vi "Get Color Icon from Caller.vi"() -> (3 "color":T1)   [LabVIEW 2021]
uses:
  <vilib>/picture/picture.llb/imagedata.ctl
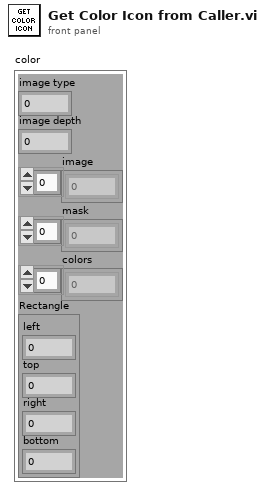
[diagram p1: front panel]
types:
  T1 = typedef "imagedata.ctl" = cluster{"image type":i32, "image depth":i32, "image":u8[], "mask":u8[], "colors":u32[], "Rectangle":cluster{"left":i16, "top":i16, "right":i16, "bottom":i16}}
  T2 = typedef "Who Invoked Icon Editor.ctl" = cluster{"Icon Editor Invoker Type":T3, "App Refnum of Invoker":refnum<vi>, "Qualified Name of Invoker":string, "Path to Invoker":path}
  T3 = typedef "Icon Editor Invoker Type.ctl" = enum32{"Unknown Icon Source", "VI Icon", "Library Icon (any library type)", "Palette icon", "Icon from App Method"}
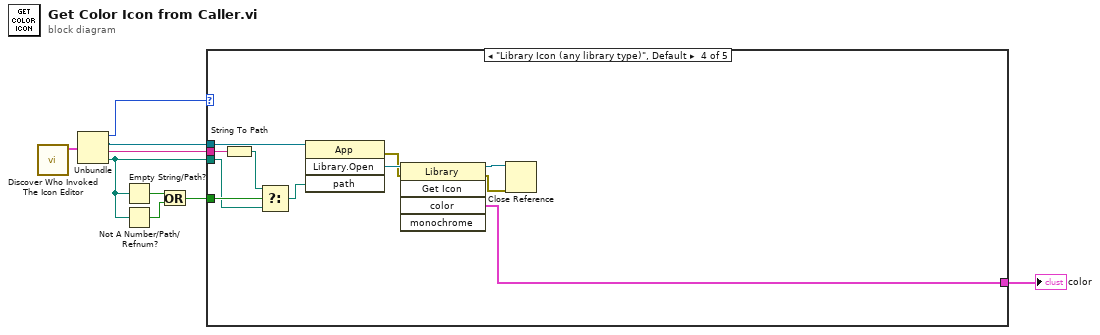
[diagram p0: block diagram]
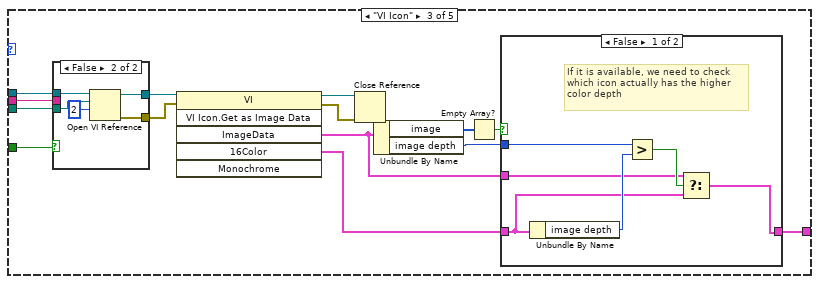
[diagram p4: hidden frame]
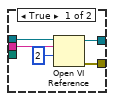
[diagram p6: hidden frame]
diagram:
  n1 = call <resource>:"Discover Who Invoked The Icon Editor.vi"() -> ("Who Invoked The Icon Editor?"=w9:T2)  [unwired: 11 out]
  n2 = Unbundle(w9) -> ("Icon Editor Invoker Type"=w7:T3, "App Refnum of Invoker"=w8:refnum<vi>, "Qualified Name of Invoker"=w3:string, "Path to Invoker"=w2:path)
  n3 = Empty String/Path?(string/path=w2) -> (empty?=w6:bool)
  n4 = Not A Number/Path/Refnum?(number/path/refnum=w2) -> (NaN/Path/Refnum?=w5:bool)
  n5 = Or(x=w6, y=w5) -> (x .or. y?=w4:bool)
  n6 = case shown="\"Library Icon (any library type)\", Default" w7 {
    tunnel: w8 -> [_ _ w21 w49 _]
    tunnel: w3 -> [_ _ w19 w45 _]
    tunnel: w2 -> [_ _ w18 w46 _]
    tunnel: w4 -> [_ _ w20 w47 _]
    tunnel: [_ _ w13 w41 _] -> w1
    frame "Unknown Icon Source" {
    }
    frame "Icon from App Method" {
    }
    frame "VI Icon" {
      n7 = case shown="False" w20 {
        tunnel: [w35 w40] -> w23
        tunnel: [w34 w39] -> w22
        tunnel: w21 -> [w33 w38]
        tunnel: w19 -> [w32 _]
        tunnel: w18 -> [_ w37]
        frame True {
          n8 = Open VI Reference(application reference (local)=w33, vi path=w32, options=2) -> (vi reference=w35:refnum<vi>, error out=w34:errorcluster)  [unwired: 1 in, 2 out]
        }
        frame False {
          n9 = Open VI Reference(application reference (local)=w38, vi path=w37, options=2) -> (vi reference=w40:refnum<vi>, error out=w39:errorcluster)  [unwired: 1 in, 2 out]
        }
      }
      n10 = invoke class="VI" method="VI Icon.Get as Image Data"(reference=w23, error in=w22) -> (reference out=w17:refnum<vi>, error out=w16:errorcluster, "ImageData"=w10:T1, "16Color"=w12:T1)  [unwired: 4 in, 2 out]
      n11 = Close Reference(reference=w17, error in (no error)=w16) -> ()  [unwired: 1 out]
      n12 = Unbundle By Name(w10) -> ("image"=w15:u8[], "image depth"=w11:i32)
      n13 = Empty Array?(array=w15) -> (empty?=w14:bool)
      n14 = case shown="False" w14 {
        tunnel: [w24 w30] -> w13
        tunnel: w12 -> [w25 w30]
        tunnel: w11 -> [w29 _]
        tunnel: w10 -> [w26 _]
        frame False {
          # "If it is available, we need to check\nwhich icon actually has the higher\ncolor depth"
          n15 = Unbundle By Name(w25) -> ("image depth"=w28:i32)
          n16 = Greater?(x=w29, y=w28) -> (0:w27:bool)
          n17 = Select(t=w26, s=w27, f=w25) -> (s? t:f=w24:T1)
        }
        frame True {
          # "Dont event bother checking\nthe 16 color icon. If it is empty\nthen we just conclude that there\nis no color icon available"
        }
      }
    }
    frame "Library Icon (any library type)", Default {
      n18 = String To Path(string=w45) -> (path=w44:path)
      n19 = Select(t=w44, s=w47, f=w46) -> (s? t:f=w43:path)
      n20 = invoke class="App" method="Library.Open"(reference=w49, "path"=w43) -> (error out=w48:errorcluster, "Open Library"=w51:refnum<vi>)  [unwired: 2 in, 2 out]
      n21 = invoke class="Library" method="Get Icon"(reference=w51, error in=w48) -> (reference out=w50:refnum<vi>, error out=w42:errorcluster, "color"=w41:T1)  [unwired: 3 in, 2 out]
      n22 = Close Reference(reference=w50, error in (no error)=w42) -> ()  [unwired: 1 out]
    }
    frame "Palette icon" {
    }
  }
  "color" <- w1
